vi "NCS_IQ_TwoTx.vi"(4 "error in":errorcluster, 5 "Coerced IQ rate":dbl, 6 "Waveform Size":dbl, 7 "Channel 1\nTone Frequency":dbl, 8 "Channel 1\nTone Amplitude":dbl, 9 "Channel 0\nTone Frequency":dbl, 10 "Channel 0\nTone Amplitude":dbl) -> (0 "error out":errorcluster, 2 "IQ waveform array":cdb[][](array[numeric]), 3 "IQ waveform":waveform(dbl)[](array[waveform]))   [LabVIEW 2016]
uses:
  <vilib>/measure/NI_MABase.lvlib
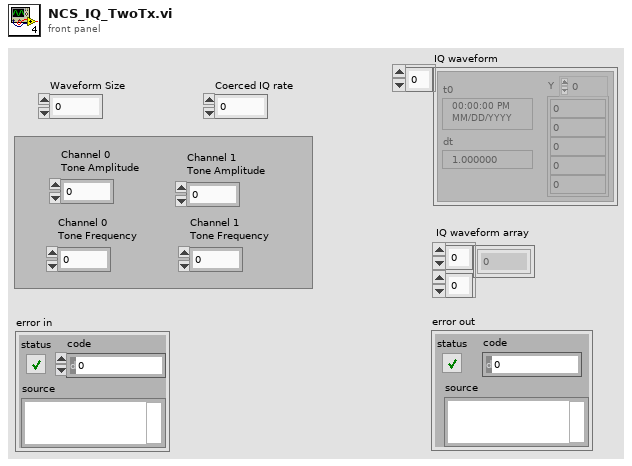
[diagram p1: front panel]
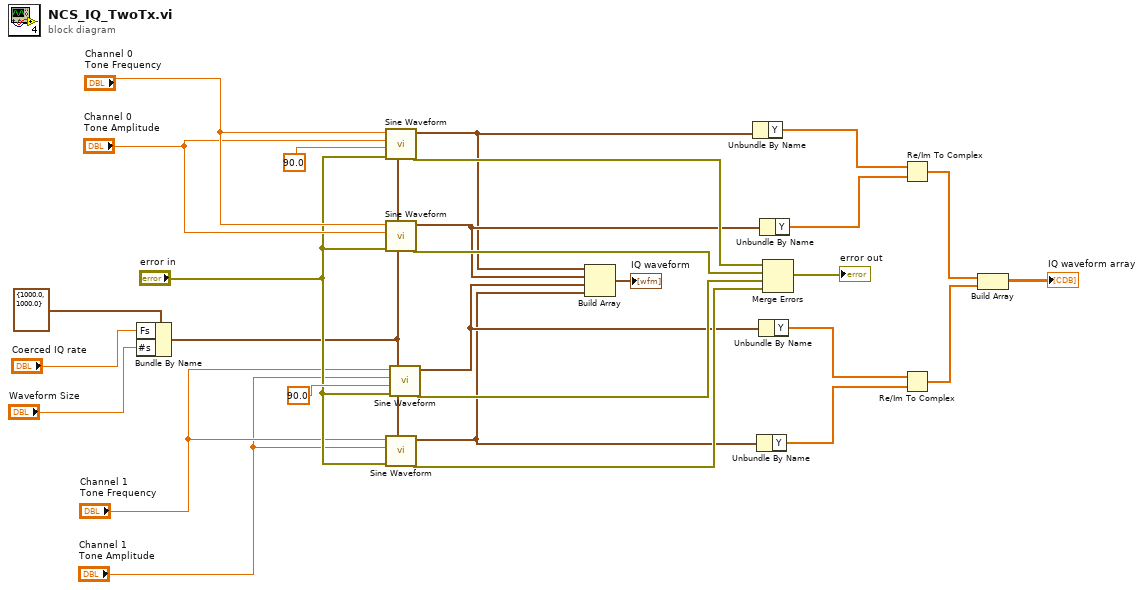
[diagram p0: block diagram]
diagram:
  n1 = Bundle By Name(cluster=cluster{"Fs":dbl, "#s":dbl} {"Fs"=1000.0, "#s"=1000.0} ("sampling info"), "Fs"="Coerced IQ rate", "#s"="Waveform Size") -> (w9:cluster{"Fs":dbl, "#s":dbl})
  n2 = call <vilib>:"Sine Waveform.vi"("sampling info"=w9, "error in (no error)"="error in", "phase"=90.0, "amplitude"="Channel 0\nTone Amplitude", "frequency"="Channel 0\nTone Frequency") -> ("error out"=w25:errorcluster, "signal out"=w16:waveform(dbl))  [unwired: 5 in]
  n3 = call <vilib>:"Sine Waveform.vi"("sampling info"=w9, "error in (no error)"="error in", "amplitude"="Channel 0\nTone Amplitude", "frequency"="Channel 0\nTone Frequency") -> ("error out"=w24:errorcluster, "signal out"=w17:waveform(dbl))  [unwired: 6 in]
  n4 = call <vilib>:"Sine Waveform.vi"("sampling info"=w9, "error in (no error)"="error in", "amplitude"="Channel 1\nTone Amplitude", "frequency"="Channel 1\nTone Frequency") -> ("error out"=w6:errorcluster, "signal out"=w1:waveform(dbl))  [unwired: 6 in]
  n5 = call <vilib>:"Sine Waveform.vi"("sampling info"=w9, "error in (no error)"="error in", "phase"=90.0, "amplitude"="Channel 1\nTone Amplitude", "frequency"="Channel 1\nTone Frequency") -> ("error out"=w11:errorcluster, "signal out"=w2:waveform(dbl))  [unwired: 5 in]
  n6 = Build Array(w16, w17, w2, w1) -> (→"IQ waveform":waveform(dbl)[])
  n7 = Unbundle By Name(w16) -> ("Y"=w20:dbl[])
  n8 = Unbundle By Name(w1) -> ("Y"=w14:dbl[])
  n9 = Unbundle By Name(w2) -> ("Y"=w13:dbl[])
  n10 = Unbundle By Name(w17) -> ("Y"=w21:dbl[])
  n11 = Merge Errors(w25, w24, w11, w6) -> (→"error out":errorcluster)
  n12 = Re/Im To Complex(1:w21, 2:w20) -> (0:w5:cdb[])
  n13 = Re/Im To Complex(1:w14, 2:w13) -> (0:w4:cdb[])
  n14 = Build Array(w5, w4) -> (→"IQ waveform array":cdb[][])
